vi "Decode HP34970A (34905A) Position2023.vi"(0 "Position to Decode":i16=1 min=0 max=5080, 1 "Total Number of Switchers":i8=1 min=0, 2 "Number of Cards in Switcher":i8=1 min=0 max=5, 3 "Last Card Used for Isolation":bool) -> (4 "ERROR - Position Out of Range":bool, 5 "Switcher":i8=1 min=1 max=21 step=1, 6 "Slot (Card)":i8=1 min=1 max=5 step=1, 7 "Group":i8 min=0 max=1, 8 "Channel":i8 min=0 max=3 step=1)   [LabVIEW 2023]
doc: "Decodes the requested position number into 4 separate lines, as required to OPEN/CLOSE a specific relay:\n\nSwitcher, Slot (Card), Group, and Channel.\n\nCurrently supports:\n\nHP3488A (44472A)"
panel:
  # "Results"
  # "Settings"
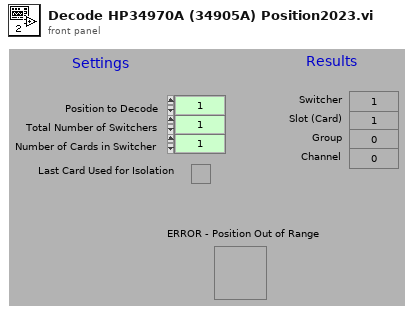
[diagram p1: front panel]
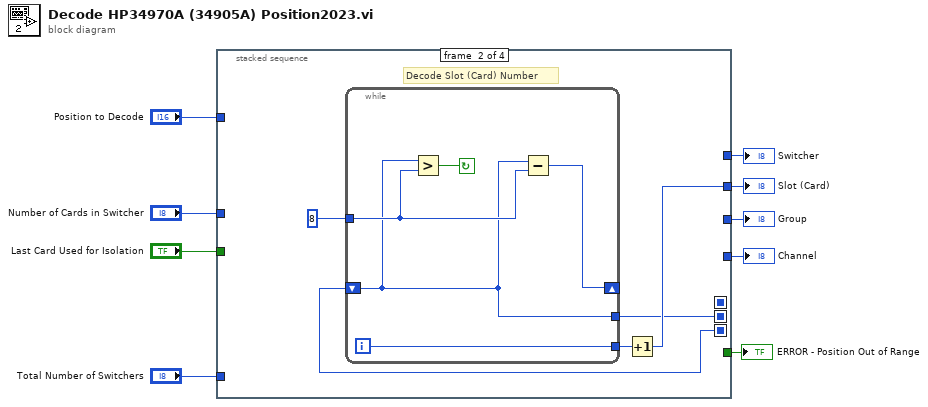
[diagram p0: block diagram]
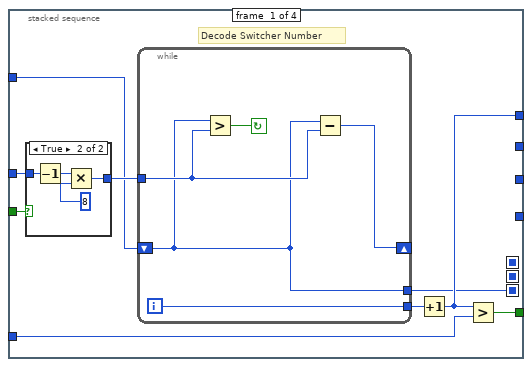
[diagram p2: hidden frame]
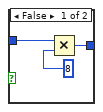
[diagram p3: hidden frame]
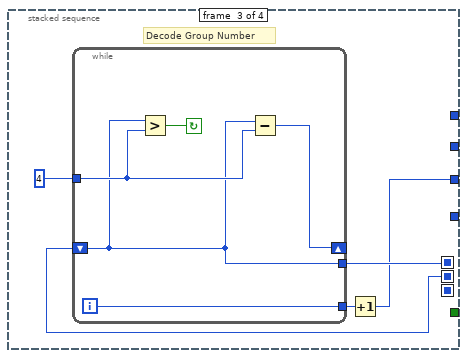
[diagram p4: hidden frame]
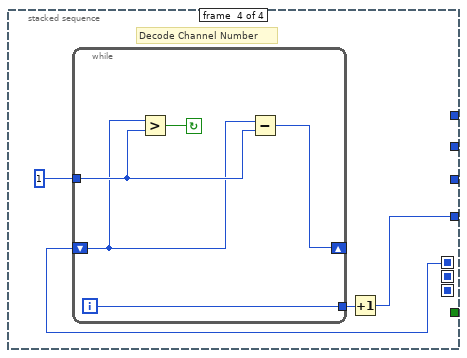
[diagram p5: hidden frame]
diagram:
  n1 = stacked-sequence {
    seq-local: [w11 _ _ _] -> [_ w33 _ _]
    seq-local: [_ w31 _ _] -> [_ _ w44 _]
    seq-local: [_ _ w43 _] -> [_ _ _ w53]
    tunnel: "Total Number of Switchers" -> [w13 _ _ _]
    tunnel: "Number of Cards in Switcher" -> [w18 _ _ _]
    tunnel: "Last Card Used for Isolation" -> [w10 _ _ _]
    tunnel: "Position to Decode" -> [w16 _ _ _]
    tunnel: [w14 _ _ _] -> w5
    tunnel: [w12 _ _ _] -> w4
    tunnel: [_ w32 _ _] -> w3
    tunnel: [_ _ w41 _] -> w2
    tunnel: [_ _ _ w51] -> w1
    frame #0 {
      # "Decode Switcher Number"
      n2 = case shown="True" w10 {
        tunnel: [w26 w30] -> w17
        tunnel: w18 -> [w24 w28]
        frame False {
          n3 = Multiply(x=w24, y=8) -> (x*y=w26:i32)
        }
        frame True {
          n4 = Decrement(x=w28) -> (x-1=w27:i8)
          n5 = Multiply(x=w27, y=8) -> (x*y=w30:i32)
        }
      }
      n6 = while {
        tunnel: [w19] -> w11
        tunnel: [w20] -> w15
        shift-left: w16 -> [w19]
        shift-right: [w21] -> _
        tunnel: w17 -> [w22]
        i -> [w20]
        stop <- w23 continue-if-true
        n7 = Greater?(x=w19, y=w22) -> (0:w23:bool)
        n8 = Subtract(x=w19, y=w22) -> (x-y=w21:i32)
      }
      n9 = Increment(x=w15) -> (x+1=w14:i32)
      n10 = Greater?(x=w14, y=w13) -> (0:w12:bool)
    }
    frame #1 {
      # "Decode Slot (Card) Number"
      n11 = while {
        tunnel: [w36] -> w31
        tunnel: [w37] -> w34
        shift-left: w33 -> [w36]
        shift-right: [w38] -> _
        tunnel: 8 -> [w39]
        i -> [w37]
        stop <- w40 continue-if-true
        n12 = Greater?(x=w36, y=w39) -> (0:w40:bool)
        n13 = Subtract(x=w36, y=w39) -> (x-y=w38:i32)
      }
      n14 = Increment(x=w34) -> (x+1=w32:i32)
    }
    frame #2 {
      # "Decode Group Number"
      n15 = while {
        tunnel: [w46] -> w43
        tunnel: [w47] -> w42
        shift-left: w44 -> [w46]
        shift-right: [w48] -> _
        tunnel: 4 -> [w49]
        i -> [w47]
        stop <- w50 continue-if-true
        n16 = Greater?(x=w46, y=w49) -> (0:w50:bool)
        n17 = Subtract(x=w46, y=w49) -> (x-y=w48:i32)
      }
      n18 = Increment(x=w42) -> (x+1=w41:i32)
    }
    frame #3 {
      # "Decode Channel Number"
      n19 = while {
        tunnel: [w56] -> w52
        shift-left: w53 -> [w55]
        shift-right: [w57] -> _
        tunnel: 1 -> [w58]
        i -> [w56]
        stop <- w59 continue-if-true
        n20 = Greater?(x=w55, y=w58) -> (0:w59:bool)
        n21 = Subtract(x=w55, y=w58) -> (x-y=w57:i32)
      }
      n22 = Increment(x=w52) -> (x+1=w51:i32)
    }
  }
  "Slot (Card)" <- w3
  "Group" <- w2
  "Channel" <- w1
  "Switcher" <- w5
  "ERROR - Position Out of Range" <- w4
